vi "Tell Arbitrary.vi"(4 "Priority":bool, 7 "Actor in":refnum<class "Actor.lvclass">, 8 "Error in":errorcluster, 9 "Transport":refnum<class "Transport.lvclass">, 10 "Msg":refnum<class "Msg.lvclass">) -> (0 "Error out":errorcluster, 5 "Actor out":refnum<class "Actor.lvclass">)   [LabVIEW 2020, in "jettl.lvlib"]
uses:
  jettl.lvlib
  Relation.ctl
  Teller Elements.ctl
  Read Self Attributes/Read Self Attributes.lvlib
  Read Self Attributes/UID.vi
  Read Self Attributes/Alias.vi
  Msg/Msg.lvclass
  Actor/Actor.lvclass
  Transport/Transport.lvclass
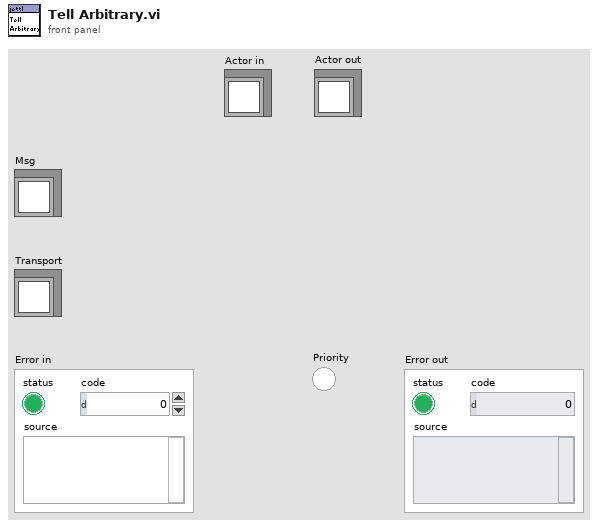
[diagram p1: front panel]
types:
  T1 = typedef "jettl.lvlib/Relation.ctl" = enum16{"Self", "Parent", "Child"}
  T2 = typedef "jettl.lvlib/Teller Elements.ctl" = cluster{"Priority":bool, "Relative Seconds":dbl, "UID":i32, "Alias":string, "Valid Relation":bool, "Relation":T1, "Told Alias":string, "Called From Msg Library":bool}
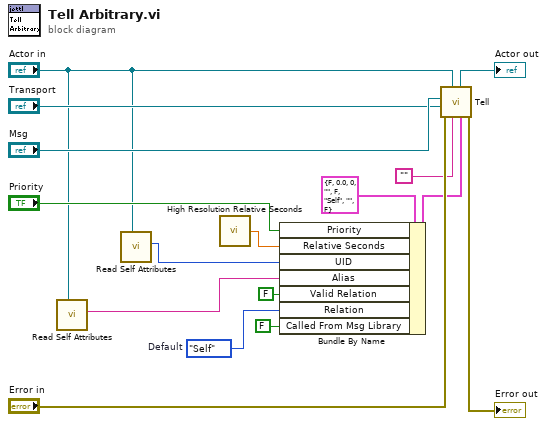
[diagram p0: block diagram]
diagram:
  w7 = Relation."Self"  # Default
  n1 = call-poly "Read Self Attributes.vi"("Actor in"="Actor in") -> ("Alias"=w4:string)  [unwired: 10 in]
  n2 = call-poly "Read Self Attributes.vi"("Actor in"="Actor in") -> ("UID"=w16:i32)  [unwired: 10 in]
  n3 = call <vilib>:"High Resolution Relative Seconds.vi"() -> ("relative seconds"=w10:dbl)
  n4 = Bundle By Name(cluster=T2 {"Priority"=FALSE, "Relative Seconds"=0.0, "UID"=0, "Alias"="", "Valid Relation"=FALSE, "Relation"=enum."Self", "Told Alias"="", "Called From Msg Library"=FALSE} ("Teller Elements"), "Priority"="Priority", "Relative Seconds"=w10, "UID"=w16, "Alias"=w4, "Valid Relation"=FALSE, "Relation"=w7, "Called From Msg Library"=FALSE) -> (w2:T2)
  n5 = call "Tell.vi"("Teller Elements"=w2, "Alias"="", "Actor in"="Actor in", "Error in"="Error in", "Transport"="Transport", "Msg"="Msg") -> ("Error out"=→"Error out":errorcluster, "Actor out"=→"Actor out":refnum<class "Actor.lvclass">)  [unwired: 4 in]
